vi "numericKeyPad.vi"() -> ()   [LabVIEW 2017]
panel:
  in  "stop":bool
  out "Entry":string
  in  "Number Keypad":T1
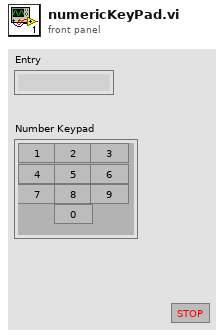
[diagram p1: front panel]
types:
  T1 = cluster{"Zero":bool, "One":bool, "Two":bool, "Three":bool, "Four":bool, "Five":bool, "Six":bool, "Seven":bool, "Eight":bool, "Nine":bool}
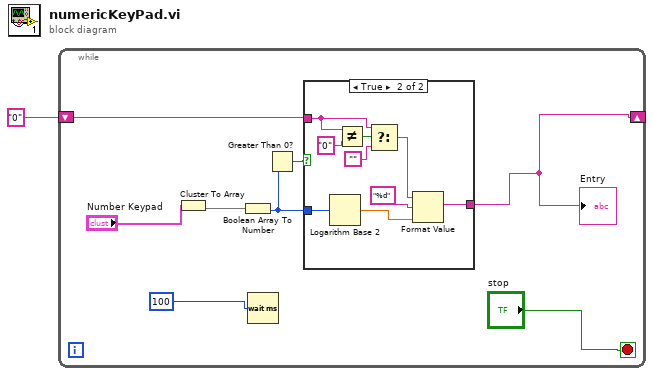
[diagram p0: block diagram]
diagram:
  n1 = while {
    shift-right: [w4] -> _
    shift-left: "0" -> [w5]
    stop <- "stop" stop-if-true
    n2 = Cluster To Array(cluster="Number Keypad") -> (array=w6:bool[])
    n3 = Boolean Array To Number(Boolean array=w6) -> (number=w3:u32)
    n4 = Wait (ms)(milliseconds to wait=u32 100) -> ()  [unwired: 1 out]
    n5 = Greater Than 0?(x=w3) -> (x > 0?=w2:bool)
    n6 = case shown="True" w2 {
      tunnel: w3 -> [_ w19]
      tunnel: w5 -> [w10 w14]
      tunnel: [w10 w17] -> w4
      frame False {
      }
      frame True {
        n7 = Logarithm Base 2(1:w19) -> (0:w11:dbl)
        n8 = Not Equal?(x=w14, y="0") -> (x != y?=w15:bool)
        n9 = Select(t=w14, s=w15, f="") -> (s? t:f=w12:string)
        n10 = Format Value(string ("")=w12, format string="%d", value (0)=w11) -> (output string=w17:string)
      }
    }
    "Entry" <- w4
  }
